vi "I2C Get Num Channels.vi"(11 "error in (no error)":errorcluster) -> (4 "numChannels out":u32, 15 "error out":errorcluster)   [LabVIEW 2017, in "libMPSSE.lvlib"]
doc: "FTDI_API FT_STATUS I2C_GetNumChannels(uint32 *numChannels);"
uses:
  libMPSSE.lvlib
  \\Mac\Home/Desktop/libMPSSE-SPI-LabVIEW-master/libMPSSE.dll
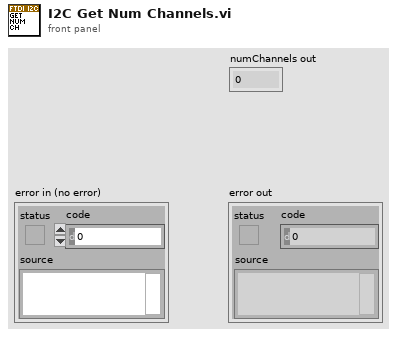
[diagram p1: front panel]
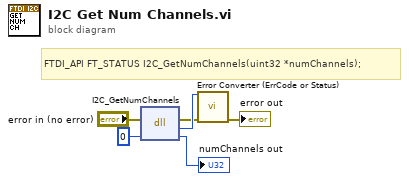
[diagram p0: block diagram]
diagram:
  # "FTDI_API FT_STATUS I2C_GetNumChannels(uint32 *numChannels);"
  n1 = dll-call lib="\\\\Mac\\Home/Desktop/libMPSSE-SPI-LabVIEW-master/libMPSSE.dll" fn="I2C_GetNumChannels"(error in="error in (no error)", "numChannels"=u32 0) -> (error out=w2:errorcluster, "return type"=w6:u32, "numChannels"=→"numChannels out":u32)  [unwired: 2 in, 1 out]
  n2 = call "Error Converter (ErrCode or Status).vi"("error code"=w6, "error in (no error)"=w2) -> ("error out"=→"error out":errorcluster)  [unwired: 13 in]
